vi "Set Gas Concentration.vi"(8 "error in (no error)":errorcluster, 10 "Gas Concentration":T1 {"Concentration" min=0.0 step=1.0}, 11 "Vapour Generator in":refnum<class "Vapour Generator.lvclass">) -> (0 "error out":errorcluster, 3 "Vapour Generator out":refnum<class "Vapour Generator.lvclass">)   [LabVIEW 2011, in "Vapour Generator.lvclass"]
uses:
  Vapour Generator.lvclass
  Gas Concentration.ctl
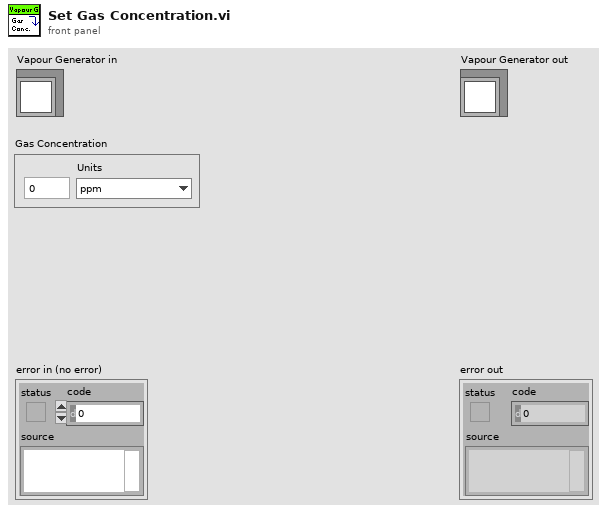
[diagram p1: front panel]
types:
  T1 = typedef "Vapour Generator.lvclass/Gas Concentration.ctl" = cluster{"Units":enum16{"ppm", "ppb", "ppt"}, "Concentration":dbl}
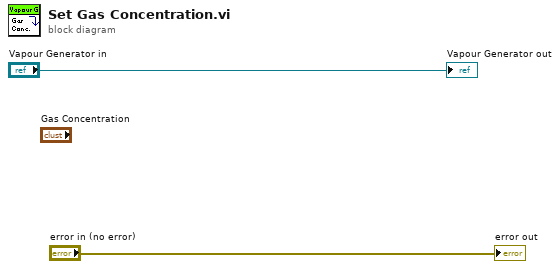
[diagram p0: block diagram]
diagram:
  "error out" <- "error in (no error)"
  "Vapour Generator out" <- "Vapour Generator in"
